vi "S2C_ProcessMenu.vi"(8 "Error In":errorcluster, 9 "Position":T1, 10 "ItemTag":string, 11 "CtlRef":refnum<vi>) -> (0 "Error Out":errorcluster)   [LabVIEW 2015]
doc: "Updates the script build table in accordance with the selected menu item."
uses:
  <vilib>/Utility/miscctls.llb/LVRowAndColumnTypeDef.ctl
  Globals/S2C_GlobalMenus.vi
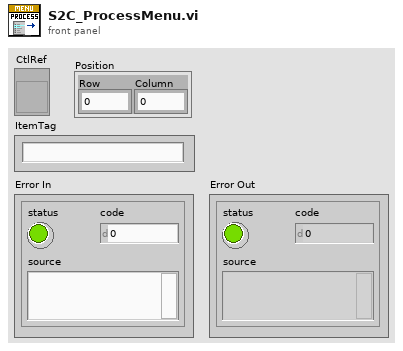
[diagram p1: front panel]
types:
  T1 = typedef "LVRowAndColumnTypeDef.ctl" = cluster{"Row":i32, "Column":i32}
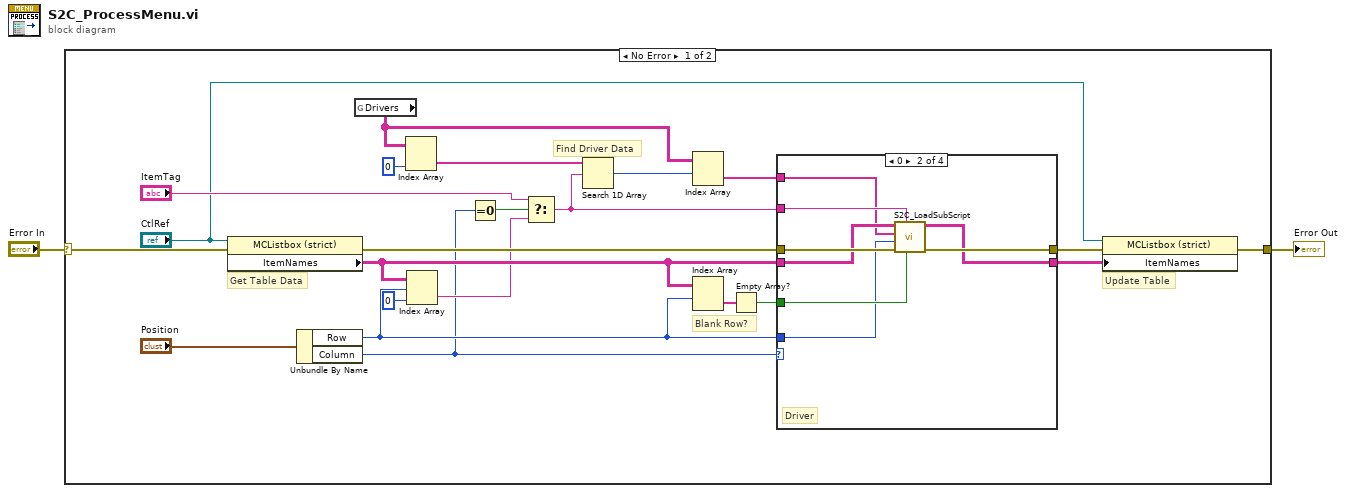
[diagram p0: block diagram]
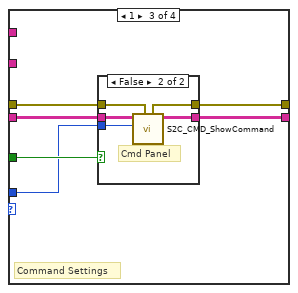
[diagram p3: hidden frame]
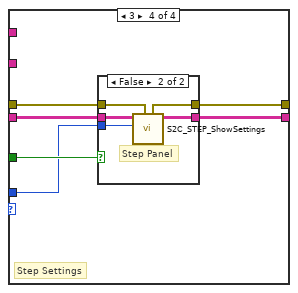
[diagram p5: hidden frame]
diagram:
  n1 = case shown="No Error" "Error In" {
    selector: "Error In" -> [w16 w61]
    tunnel: [w4 w61] -> w1
    frame No Error {
      # "Update Table"
      # "Get Table Data"
      # "Find Driver Data"
      # "Blank Row?"
      n2 = property on="Property Node" class="MCListbox (strict)"(reference="CtlRef", error in=w16) -> (error out=w23:errorcluster, "ItemNames"=w14:string[][])  [unwired: 1 out]
      n3 = Unbundle By Name("Position") -> ("Row"=w13:i32, "Column"=w7:i32)
      n4 = global read "S2C_GlobalMenus.vi" "Drivers"() -> (w18:string[][])
      n5 = Index Array(array=w18, index (col)=0 ("disabled index (col)")) -> (element=w20:string[])  [unwired: 1 in]
      n6 = Index Array(array=w14, index (row)=w13, index (col)=0 ("disabled index (col)")) -> (element=w9:string)
      n7 = Equal To 0?(x=w7) -> (x = 0?=w11:bool)
      n8 = Select(t="ItemTag", s=w11, f=w9) -> (s? t:f=w8:string)
      n9 = Search 1D Array(1D array=w20, element=w8) -> (index of element=w19:i32)  [unwired: 1 in]
      n10 = Index Array(array=w18, index (row)=w19) -> (element=w15:string[])  [unwired: 1 in]
      n11 = Index Array(array=w14, index (row)=w13) -> (element=w24:string[])  [unwired: 1 in]
      n12 = Empty Array?(array=w24) -> (empty?=w22:bool)
      n13 = case shown="0" w7 {
        tunnel: w15 -> [_ w27 _ _]
        tunnel: [w25 w31 w40 w53] -> w5
        tunnel: w14 -> [w25 w32 w39 w52]
        tunnel: w22 -> [_ w30 w38 w51]
        tunnel: w23 -> [w26 w34 w37 w50]
        tunnel: [w26 w33 w36 w49] -> w6
        tunnel: w13 -> [_ w28 w35 w48]
        tunnel: w8 -> [_ w29 _ _]
        frame -1, Default {
          # "Undefined Column"
        }
        frame 0 {
          # "Driver"
          n14 = call "S2C_LoadSubScript.vi"("Insert?"=w30, "ItemTag"=w29, "Error In"=w34, "Row"=w28, "FuncData"=w27, "TblData In"=w32) -> ("Error Out"=w33:errorcluster, "TblData Out"=w31:string[][])  [unwired: 4 in]
        }
        frame 1 {
          # "Command Settings"
          n15 = case shown="False" w38 {
            tunnel: [w41 w46] -> w40
            tunnel: w39 -> [w41 w47]
            tunnel: w37 -> [w42 w45]
            tunnel: [w42 w44] -> w36
            tunnel: w35 -> [_ w43]
            frame True {
              # "Blank Row"
            }
            frame False {
              # "Cmd Panel"
              n16 = call "S2C_CMD_ShowCommand.vi"("Error In"=w45, "Row"=w43, "Data In"=w47) -> ("Data Out"=w46:string[][], "Error Out"=w44:errorcluster)  [unwired: 7 in]
            }
          }
        }
        frame 3 {
          # "Step Settings"
          n17 = case shown="False" w51 {
            tunnel: [w54 w59] -> w53
            tunnel: w52 -> [w54 w60]
            tunnel: w50 -> [w55 w57]
            tunnel: [w55 w56] -> w49
            tunnel: w48 -> [_ w58]
            frame True {
              # "Blank Row"
            }
            frame False {
              # "Step Panel"
              n18 = call "S2C_STEP_ShowSettings.vi"("Error In"=w57, "Row"=w58, "Data In"=w60) -> ("Data Out"=w59:string[][], "Error Out"=w56:errorcluster)  [unwired: 7 in]
            }
          }
        }
      }
      n19 = property class="MCListbox (strict)"(reference="CtlRef", error in=w6, "ItemNames"=w5) -> (error out=w4:errorcluster)  [unwired: 1 out]
    }
    frame Error {
    }
  }
  "Error Out" <- w1
